vi "Calc Close the Loop Params.vi"(9 "P_toolf":dbl[](array[numeric]), 10 "a_67f":dbl[](array[numeric]), 11 "S_6f":dbl[](array[numeric])) -> (0 "a_71":dbl, 1 "alpha_71":dbl, 2 "theta_7":dbl, 3 "gamma_1":dbl, 4 "S_1":dbl, 5 "S_7":dbl)   [LabVIEW 2017, in "NI_Robotics_Analytical Serial Arm Class.lvclass"]
uses:
  <vilib>/robotics/Kinematics/Analytical/Generic/NI_Robotics_Analytical Serial Arm Class.lvclass
  <vilib>/Analysis/_algsub.llb/Real Vector Norm.vi
  <vilib>/Analysis/baseanly.llb/Real Dot Product.vi
  <vilib>/Analysis/NI_AALPro.lvlib
  <vilib>/Analysis/NI_AALBase.lvlib
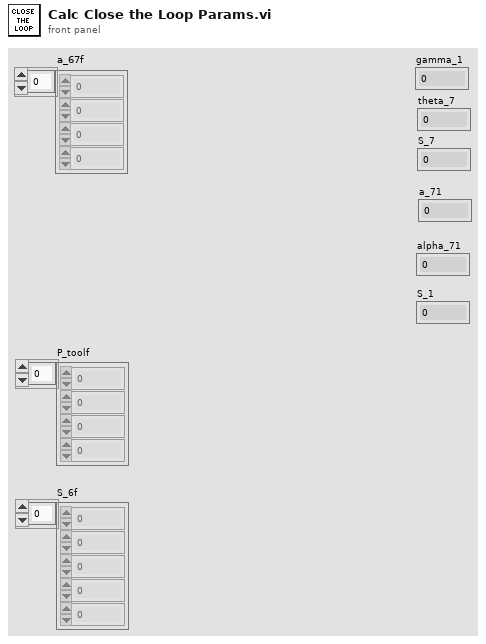
[diagram p1: front panel]
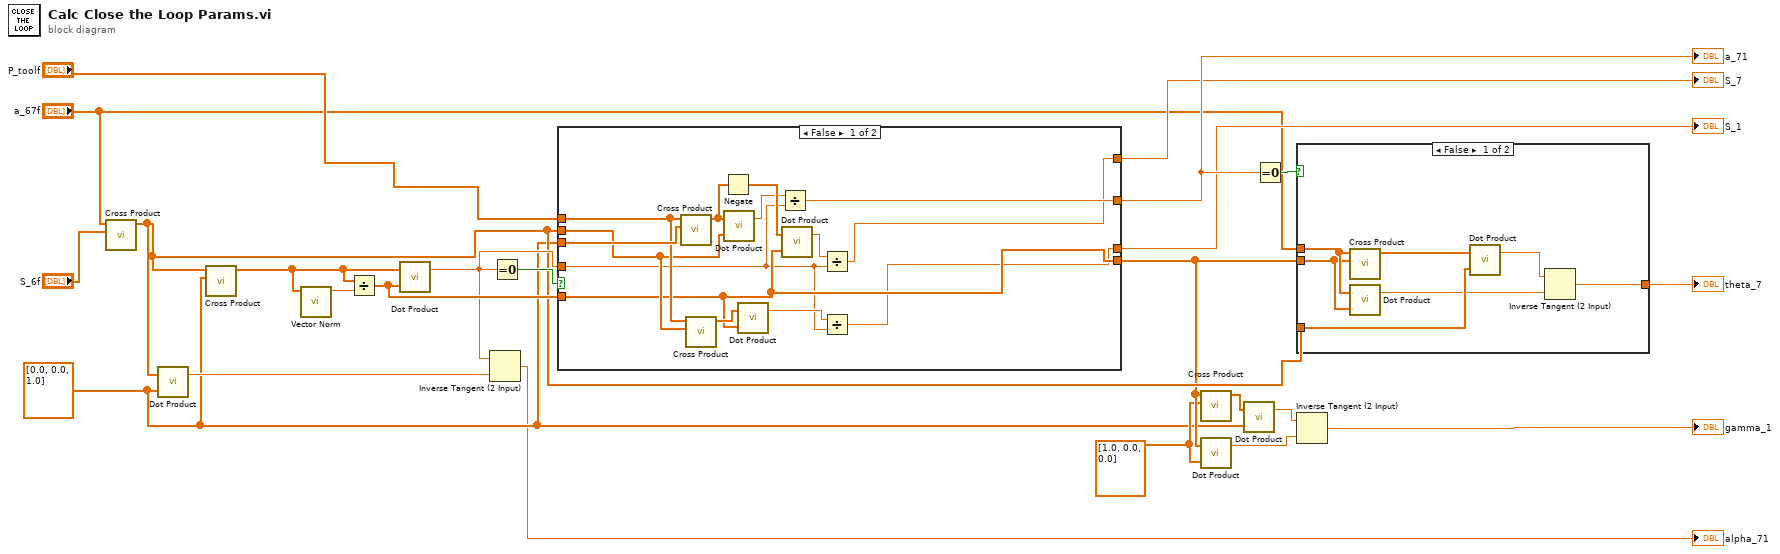
[diagram p0: block diagram]
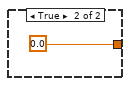
[diagram p2: hidden frame]
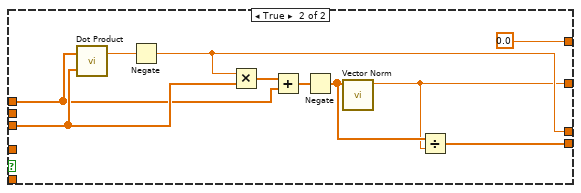
[diagram p3: hidden frame]
diagram:
  w13 = dbl[] [1.0, 0.0, 0.0]
  w11 = dbl[] [0.0, 0.0, 1.0]
  n1 = call <vilib>:"Cross Product.vi"("B Vector"="S_6f", "A Vector"="a_67f") -> ("Cross Product"=w15:dbl[])  [unwired: 8 in, 1 out]
  n2 = call-poly <vilib>:"Dot Product.vi"("Y Vector"=w11, "X Vector"=w15) -> ("X * Y"=w21:dbl)  [unwired: 1 out]
  n3 = call <vilib>:"Cross Product.vi"("B Vector"=w11, "A Vector"=w15) -> ("Cross Product"=w22:dbl[])  [unwired: 8 in, 1 out]
  n4 = call-poly <vilib>:"Vector Norm.vi"("Input Vector"=w22) -> ("norm"=w23:dbl)  [unwired: 9 in, 1 out]
  n5 = Divide(x=w22, y=w23) -> (x/y=w19:dbl[])
  n6 = call-poly <vilib>:"Dot Product.vi"("Y Vector"=w19, "X Vector"=w22) -> ("X * Y"=w18:dbl)  [unwired: 1 out]
  n7 = Inverse Tangent (2 Input)(1:w21, 2:w18) -> (0:→"alpha_71":dbl)
  n8 = Equal To 0?(x=w18) -> (x = 0?=w20:bool)
  n9 = case shown="False" w20 {
    tunnel: "P_toolf" -> [w30 w44]
    tunnel: w11 -> [w32 w46]
    tunnel: [w24 w41] -> w5
    tunnel: [w34 w38] -> w16
    tunnel: [w27 w42] -> w14
    tunnel: [w33 0.0 ("-x")] -> w4
    tunnel: w19 -> [w27 _]
    tunnel: w15 -> [w29 _]
    tunnel: w18 -> [w25 _]
    frame False {
      n10 = call <vilib>:"Cross Product.vi"("B Vector"=w32, "A Vector"=w30) -> ("Cross Product"=w31:dbl[])  [unwired: 8 in, 1 out]
      n11 = call <vilib>:"Cross Product.vi"("B Vector"=w29, "A Vector"=w30) -> ("Cross Product"=w28:dbl[])  [unwired: 8 in, 1 out]
      n12 = Negate(x=w31) -> (-x=w37:dbl[])
      n13 = call-poly <vilib>:"Dot Product.vi"("Y Vector"=w29, "X Vector"=w31) -> ("X * Y"=w35:dbl)  [unwired: 1 out]
      n14 = call-poly <vilib>:"Dot Product.vi"("Y Vector"=w27, "X Vector"=w28) -> ("X * Y"=w26:dbl)  [unwired: 1 out]
      n15 = Divide(x=w35, y=w25) -> (x/y=w34:dbl)
      n16 = call-poly <vilib>:"Dot Product.vi"("Y Vector"=w27, "X Vector"=w37) -> ("X * Y"=w36:dbl)  [unwired: 1 out]
      n17 = Divide(x=w36, y=w25) -> (x/y=w33:dbl)
      n18 = Divide(x=w26, y=w25) -> (x/y=w24:dbl)
    }
    frame True {
      n19 = call-poly <vilib>:"Dot Product.vi"("Y Vector"=w46, "X Vector"=w44) -> ("X * Y"=w47:dbl)  [unwired: 1 out]
      n20 = Negate(x=w47) -> (-x=w41:dbl)
      n21 = Multiply(x=w41, y=w46) -> (x*y=w45:dbl[])
      n22 = Add(x=w45, y=w44) -> (x+y=w43:dbl[])
      n23 = Negate(x=w43) -> (-x=w39:dbl[])
      n24 = call-poly <vilib>:"Vector Norm.vi"("Input Vector"=w39) -> ("norm"=w38:dbl)  [unwired: 9 in, 1 out]
      n25 = Divide(x=w39, y=w38) -> (x/y=w42:dbl[])
    }
  }
  "S_1" <- w5
  "S_7" <- w4
  "a_71" <- w16
  n26 = call <vilib>:"Cross Product.vi"("B Vector"=w13, "A Vector"=w14) -> ("Cross Product"=w12:dbl[])  [unwired: 8 in, 1 out]
  n27 = call-poly <vilib>:"Dot Product.vi"("Y Vector"=w13, "X Vector"=w14) -> ("X * Y"=w9:dbl)  [unwired: 1 out]
  n28 = call-poly <vilib>:"Dot Product.vi"("Y Vector"=w11, "X Vector"=w12) -> ("X * Y"=w10:dbl)  [unwired: 1 out]
  n29 = Equal To 0?(x=w16) -> (x = 0?=w17:bool)
  n30 = case shown="False" w17 {
    tunnel: [w48 0.0] -> w7
    tunnel: "a_67f" -> [w54 _]
    tunnel: w14 -> [w53 _]
    tunnel: w15 -> [w51 _]
    frame False {
      n31 = call <vilib>:"Cross Product.vi"("B Vector"=w53, "A Vector"=w54) -> ("Cross Product"=w52:dbl[])  [unwired: 8 in, 1 out]
      n32 = call-poly <vilib>:"Dot Product.vi"("Y Vector"=w53, "X Vector"=w54) -> ("X * Y"=w49:dbl)  [unwired: 1 out]
      n33 = call-poly <vilib>:"Dot Product.vi"("Y Vector"=w51, "X Vector"=w52) -> ("X * Y"=w50:dbl)  [unwired: 1 out]
      n34 = Inverse Tangent (2 Input)(1:w49, 2:w50) -> (0:w48:dbl)
    }
    frame True {
    }
  }
  "theta_7" <- w7
  n35 = Inverse Tangent (2 Input)(1:w9, 2:w10) -> (0:→"gamma_1":dbl)
